vi "Unzip VIPM Package.vi"(8 "error in (no error)":errorcluster, 11 "Source VIPM package (.vip)":path) -> (0 "error out":errorcluster, 3 "VIPM package spec filepath":path)   [LabVIEW 2014, in "vipm-to-nipm-package-converter.lvlib"]
doc: "Unzips VIPM package and returns the spec filepath"
uses:
  vipm-to-nipm-package-converter.lvlib
  <vilib>/Utility/sysdir.llb/System Directory Type.ctl
  <vilib>/zip/NI_Unzip.lvlib
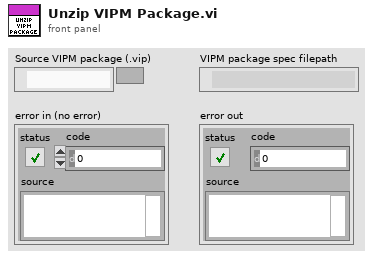
[diagram p1: front panel]
types:
  T1 = typedef "System Directory Type.ctl" = i32
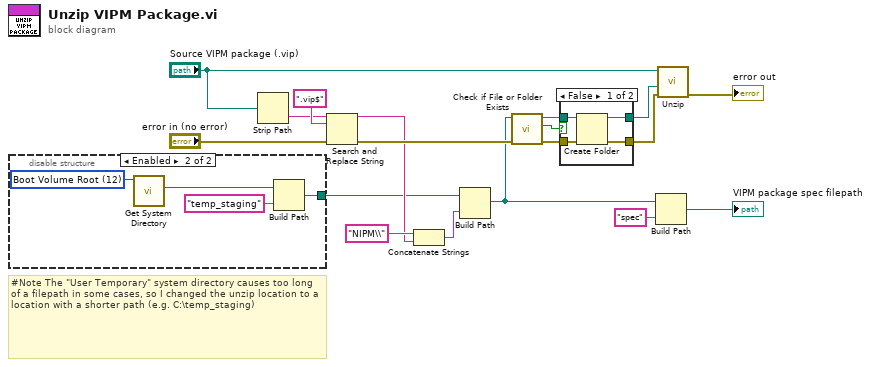
[diagram p0: block diagram]
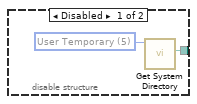
[diagram p2: hidden frame]
diagram:
  # "#Note The \"User Temporary\" system directory causes too long of a filepath in some cases, so I changed the unzip location to a location with a shorter path (e.g. C:\\temp_staging)"
  n1 = disable-structure shown="Enabled" {
    disable-tunnel: [w20 w21] -> w1
    frame Disabled {
      w19 = T1 5 items=["User Home"=0, "User Desktop"=1, "User Documents"=2, "User Application Data"=3, "User Preferences"=4, "User Temporary"=5, "Public Documents"=6, "Public Application Data"=7, "Public Preferences"=8, "Public Cache"=13, "System Core Libraries"=9, "System Installed Libraries"=10, "Application Files"=11, "Boot Volume Root"=12] ("system directory type")
      n2 = call <vilib>:"Get System Directory.vi"("system directory type"=w19) -> ("system directory"=w20:path)  [unwired: 10 in]
    }
    frame Enabled {
      w24 = T1 12 items=["User Home"=0, "User Desktop"=1, "User Documents"=2, "User Application Data"=3, "User Preferences"=4, "User Temporary"=5, "Public Documents"=6, "Public Application Data"=7, "Public Preferences"=8, "Public Cache"=13, "System Core Libraries"=9, "System Installed Libraries"=10, "Application Files"=11, "Boot Volume Root"=12] ("system directory type")
      n3 = call <vilib>:"Get System Directory.vi"("system directory type"=w24) -> ("system directory"=w23:path)  [unwired: 10 in]
      n4 = Build Path(base path=w23, name or relative path="temp_staging") -> (appended path=w21:path)
    }
  }
  n5 = Strip Path(path="Source VIPM package (.vip)") -> (name=w5:string)  [unwired: 1 out]
  n6 = Search and Replace String(input string=w5, search string=".vip$", error in="error in (no error)") -> (result string=w4:string, error out=w14:errorcluster)  [unwired: 5 in, 2 out]
  n7 = Concatenate Strings("NIPM\\" ("string"), w4) -> (w2:string)
  n8 = Build Path(base path=w1, name or relative path=w2) -> (appended path=w13:path)
  n9 = call <vilib>:"Check if File or Folder Exists.vi"("error in (no error)"=w14, "path"=w13) -> ("error out"=w15:errorcluster, "file or folder exists?"=w10:bool, "dup path"=w11:path)  [unwired: 7 in]
  n10 = case shown="False" w10 {
    tunnel: w11 -> [w28 w30]
    tunnel: [w27 w30] -> w12
    tunnel: w15 -> [w26 w29]
    tunnel: [w25 w29] -> w16
    frame False {
      n11 = Create Folder(path (use dialog)=w28, error in=w26) -> (created path=w27:path, error out=w25:errorcluster)  [unwired: 1 in, 1 out]
    }
    frame True {
    }
  }
  n12 = Build Path(base path=w13, name or relative path="spec") -> (appended path=→"VIPM package spec filepath":path)
  n13 = call <vilib>:"Unzip.vi"("error in (no error)"=w16, "Target directory (same as Zip file if empty)"=w12, "Zip file"="Source VIPM package (.vip)") -> ("error out"=→"error out":errorcluster)  [unwired: 6 in, 2 out]
